vi "Main.vi"(11 "Module Admin":refnum<class "Delacor_lib_QMH_Module Admin.lvclass">) -> ()   [LabVIEW 2019, in "Helper loop.lvlib"]
doc: "This template is based off of the Queued Message Handler design pattern and the Queued Message Handler project template that ships with LabVIEW.\n\nThe main difference is that the queue is private to this module and communication between modules is performed via Broadcast and Request events.\n\nRequest events are wrapped in public API methods and are handled in the Event Handling Loop (EHL) of this VI. Any module can register for Broadcast events sent by this module. The EHL generates messages based on user interface actions.\n\nThe Message Handling Loop (MHL) processes messages generated by the EHL, or by other messages. The messages are string values, so new messages can be added easily to the Message Cases case structure in the MHL. Each message cluster can also provide an optional value for Message Data, which is a variant that can be converted to whatever message-specific data is required.\n_____\nBased on Delacor QMH Project Template 5.0.0.82."
uses:
  Helper loop.lvlib
  Module Data--cluster.ctl
  <vilib>/Delacor/Delacor QMH/Libraries/Message Queue_class/Delacor_lib_QMH_Message Queue.lvclass
  <vilib>/Delacor/Delacor QMH/Libraries/Message Queue_class/Delacor_lib_QMH_Enqueue Message (Single).vi
  <vilib>/ErrorRing/Error Ring.xnode
  <vilib>/Utility/error.llb/Error Cluster From Error Code.vi
  Stop Argument--cluster.ctl
  <vilib>/Delacor/Delacor QMH/Libraries/Module Admin_class/Delacor_lib_QMH_Module Admin.lvclass
  <vilib>/Utility/miscctls.llb/LVPointTypeDef.ctl
  STOP_HELPER_LOOP Argument--cluster.ctl
  DQMHSUBPANE/Libraries/HELPER LOOP ACQ/HELPER LOOP ACQ.lvlib
panel:
  in  "Simulate MHL Error":bool
  in  "Simulate EHL Error":bool
  out "error out":errorcluster
  out "Status":string
  # "Other QMH Modules communicate with this Module via its Public API (wrappers for its Request Events).\n\nThis Module communicates with other Modules via its Broadcast Events.\nAny module that wants to get these messages, just registers for this module's Broadcast events."
  # "This template is for the Delacor Modified Queued Message Handler design pattern.\n\nSee the block diagram for more information on how to use this template."
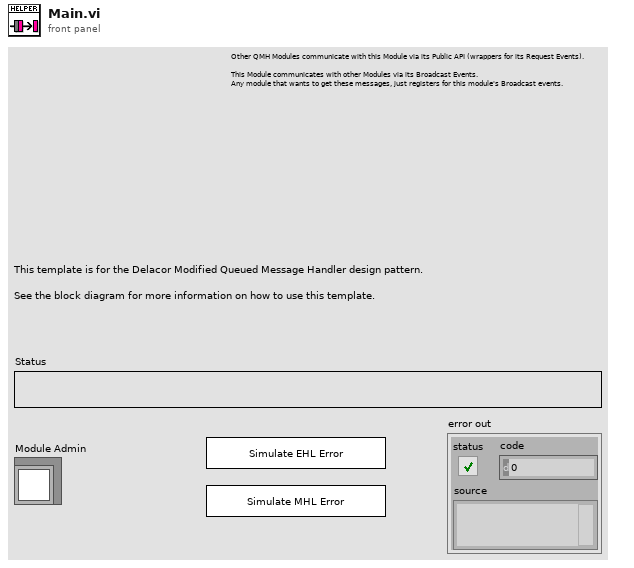
[diagram p1: front panel]
types:
  T1 = typedef "Helper loop.lvlib/Request Events--cluster.ctl" = cluster{"Stop Module":refnum<user-event>, "Show Panel":refnum<user-event>, "Hide Panel":refnum<user-event>, "Get Module Execution Status":refnum<user-event>, "Show Diagram":refnum<user-event>, "START_HELPER_LOOP":refnum<user-event>, "STOP_HELPER_LOOP":refnum<user-event>}
  T2 = typedef "Helper loop.lvlib/Module Data--cluster.ctl" = cluster{"Status":string}
  T3 = typedef "Helper loop.lvlib/STOP_HELPER_LOOP Argument--cluster.ctl" = cluster{"Boolean":bool}
  T4 = enum32{"invalid lock state", "Not Locked", "Locked (No Password)", "Password-protected"}
  T5 = typedef "Helper loop.lvlib/Stop Argument--cluster.ctl" = cluster{"Origin":string, "Exit via Stop Module Req?":bool, "Wait for Module to stop?":bool}
  T6 = typedef "LVPointTypeDef.ctl" = cluster{"Horizontal":i16, "Vertical":i16}
  T7 = enum32{"Invalid", "Standard", "Closed", "Hidden", "Minimized", "Maximized"}
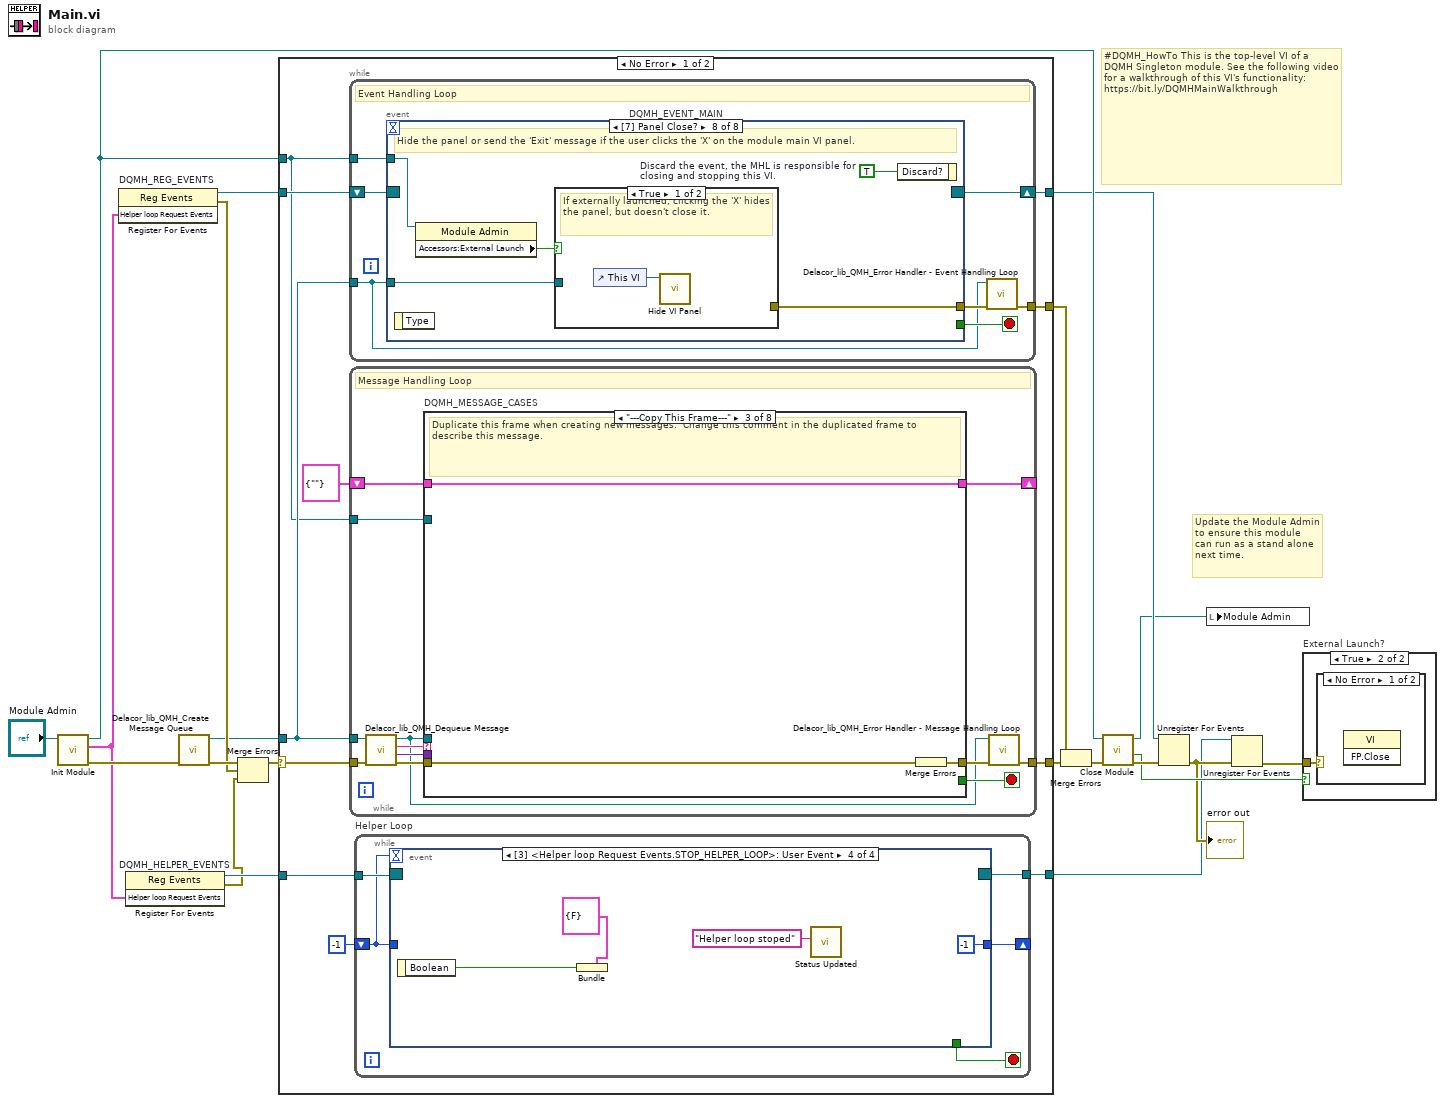
[diagram p0: block diagram]
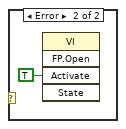
[diagram p3: hidden frame]
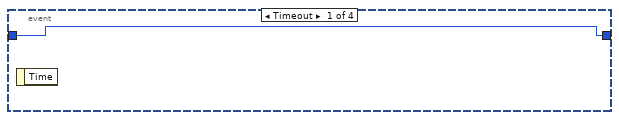
[diagram p4: hidden frame]
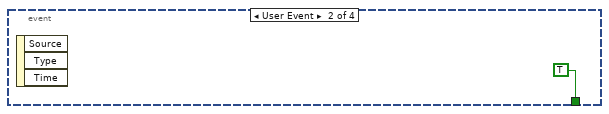
[diagram p5: hidden frame]
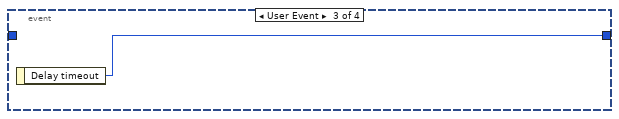
[diagram p6: hidden frame]
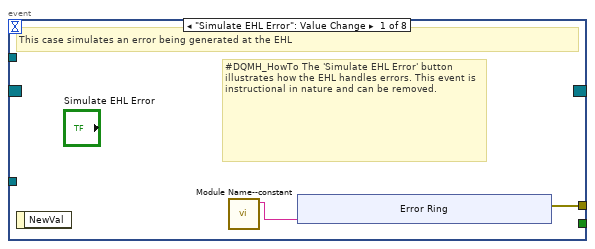
[diagram p7: hidden frame]
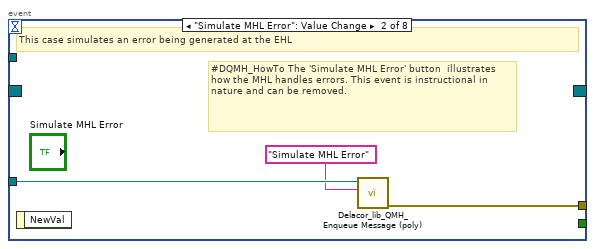
[diagram p8: hidden frame]
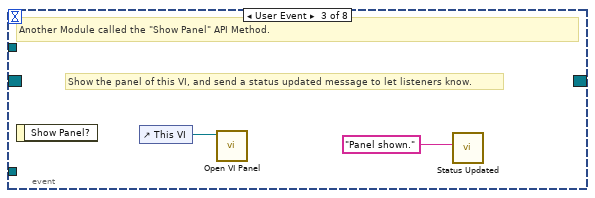
[diagram p9: hidden frame]
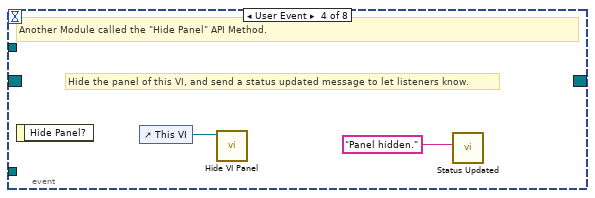
[diagram p10: hidden frame]
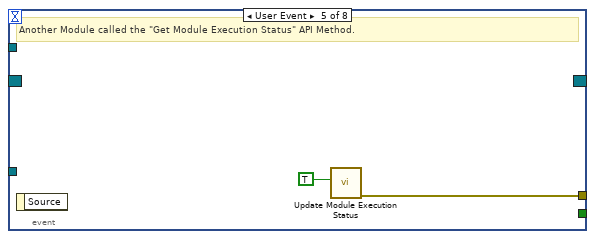
[diagram p11: hidden frame]
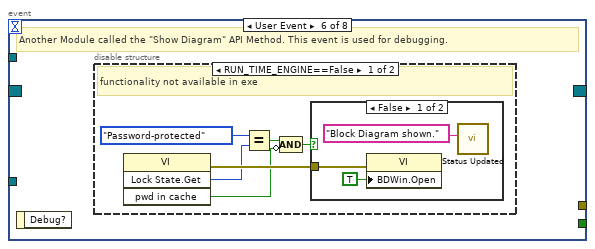
[diagram p12: hidden frame]
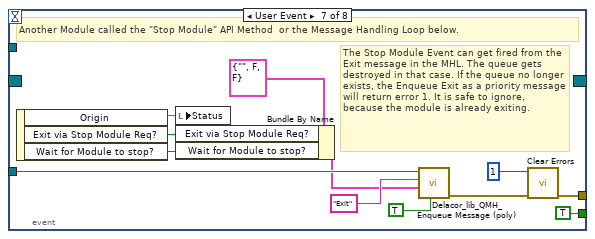
[diagram p15: hidden frame]
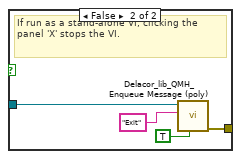
[diagram p16: hidden frame]
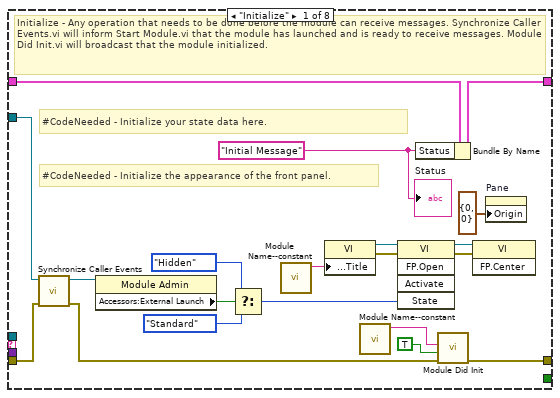
[diagram p17: hidden frame]
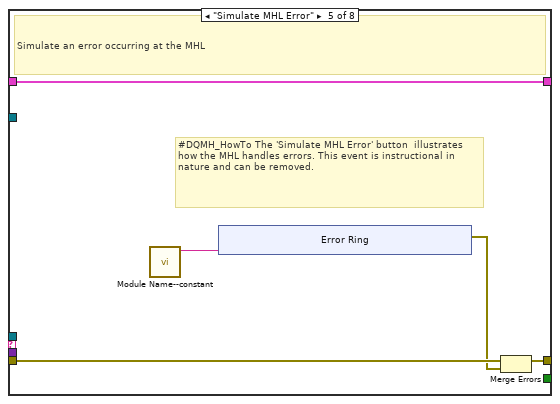
[diagram p20: hidden frame]
diagram:
  # "#DQMH_HowTo This is the top-level VI of a DQMH Singleton module. See the following video for a walkthrough of this VI's functionality: https://bit.ly/DQMHMainWalkthrough"
  # "Update the Module Admin to ensure this module can run as a stand alone next time."
  n1 = call "Init Module.vi"("Singleton Module Admin in"="Module Admin") -> ("error out"=w20:errorcluster, "Helper loop Request Events"=w6:T1, "Singleton Module Admin out"=w13:refnum<class "Delacor_lib_QMH_Module Admin.lvclass">)  [unwired: 8 in]
  n2 = register-events "DQMH_REG_EVENTS"(w6) -> (reference out=w11:refnum<event-registration>, error out=w14:errorcluster)  [unwired: 2 in]
  n3 = register-events "DQMH_HELPER_EVENTS"(w6) -> (reference out=w5:refnum<event-registration>, error out=w4:errorcluster)  [unwired: 2 in]
  n4 = call <vilib>:"Delacor_lib_QMH_Create Message Queue.vi"("error in (no error)"=w20) -> ("error out"=w16:errorcluster, "Message Queue"=w10:refnum<class "Delacor_lib_QMH_Message Queue.lvclass">)  [unwired: 9 in]
  n5 = Merge Errors(w16, w14, w4) -> (w15:errorcluster)
  n6 = case shown="No Error" w15 {
    selector: w15 -> [w30 w201]
    tunnel: [w32 w200] -> w21
    tunnel: [w29 w206] -> w12
    tunnel: w11 -> [w27 w206]
    tunnel: w10 -> [w26 w199]
    tunnel: [w31 _] -> w18
    tunnel: w13 -> [w25 w202]
    tunnel: w5 -> [w24 w198]
    tunnel: [w23 w198] -> w1
    frame No Error {
      n7 = while {
        tunnel: w26 -> [w45]
        shift-right: [w48] -> w29
        shift-left: w27 -> [w49]
        tunnel: [w50] -> w31
        tunnel: w25 -> [w46]
        stop <- w47 stop-if-true
        # "Event Handling Loop"
        n8 = event "DQMH_EVENT_MAIN" shown="[7] Panel Close?" {
          selector: w49 -> [_ _ _ _ _ _ _ _]
          dyn-events: [_ _ _ _ _ _ _ _] -> w48
          timeout: _ -> [_ _ _ _ _ _ _ _]
          tunnel: [_ _ _ _ _ _ TRUE ("Discard?") _] -> w47
          tunnel: w45 -> [_ w62 _ _ _ _ w86 w93]
          tunnel: [w53 w63 _ _ w69 _ w89 w95] -> w51
          tunnel: w46 -> [_ _ _ _ _ _ _ w92]
          event "Simulate EHL Error": Value Change {
            # "#DQMH_HowTo The 'Simulate EHL Error' button  illustrates how the EHL handles errors. This event is instructional in nature and can be removed."
            # "This case simulates an error being generated at the EHL"
            n9 = event-data() -> ()  [unwired: 1 in, 1 out]
            n10 = call "Module Name--constant.vi"() -> ("Module Name"=w52:string)  [unwired: 11 in]
            n11 = xnode "Error Ring"("parameter 0"=w52) -> ("error out"=w53:errorcluster)
          }
          event "Simulate MHL Error": Value Change {
            # "#DQMH_HowTo The 'Simulate MHL Error' button  illustrates how the MHL handles errors. This event is instructional in nature and can be removed."
            # "This case simulates an error being generated at the EHL"
            n12 = event-data() -> ()  [unwired: 1 in, 1 out]
            n13 = call-poly <vilib>:"Delacor_lib_QMH_Enqueue Message (poly).vi"("Message"="Simulate MHL Error", "Message Queue in"=w62) -> ("error out"=w63:errorcluster)  [unwired: 8 in, 1 out]
          }
          event User Event {
            # "Show the panel of this VI, and send a status updated message to let listeners know."
            # "Another Module called the \"Show Panel\" API Method."
            n14 = event-data() -> ()  [unwired: 1 in, 1 out]
            n15 = control-ref of="This VI"() -> (w65:refnum<vi>)
            n16 = call "Open VI Panel.vi"("VI"=w65) -> ()  [unwired: 10 in, 1 out]
            n17 = call "Status Updated.vi"("Status"="Panel shown." ("format string")) -> ()  [unwired: 10 in, 1 out]
          }
          event User Event {
            # "Hide the panel of this VI, and send a status updated message to let listeners know."
            # "Another Module called the \"Hide Panel\" API Method."
            n18 = event-data() -> ()  [unwired: 1 in, 1 out]
            n19 = control-ref of="This VI"() -> (w67:refnum<vi>)
            n20 = call "Hide VI Panel.vi"("VI"=w67) -> ()  [unwired: 10 in, 1 out]
            n21 = call "Status Updated.vi"("Status"="Panel hidden." ("format string")) -> ()  [unwired: 10 in, 1 out]
          }
          event User Event {
            # "Another Module called the \"Get Module Execution Status\" API Method."
            n22 = event-data() -> ()  [unwired: 1 in, 1 out]
            n23 = call "Update Module Execution Status.vi"("Running?"=TRUE) -> ("error out"=w69:errorcluster)  [unwired: 10 in]
          }
          event User Event {
            # "Another Module called the \"Show Diagram\" API Method. This event is used for debugging."
            n24 = event-data() -> ()  [unwired: 1 in, 1 out]
            n25 = disable-structure shown="RUN_TIME_ENGINE==False" {
              frame condition #0 (active) {
                # "functionality not available in exe"
                n26 = invoke class="VI" method="Lock State.Get"() -> (error out=w75:errorcluster, "Get Lock State"=w74:T4, "pwd in cache"=w71:bool)  [unwired: 4 in, 1 out]
                n27 = Equal?(x=T4."Password-protected", y=w74) -> (x = y?=w72:bool)
                n28 = Compound Arithmetic op=AND(w72, invert w71) -> (w70:bool)
                n29 = case shown="False" w70 {
                  tunnel: w75 -> [w78 _]
                  frame False {
                    n30 = property class="VI"(error in=w78, "BDWin.Open"=TRUE ("Block Diagram Window:Open")) -> ()  [unwired: 1 in, 2 out]
                    n31 = call "Status Updated.vi"("Status"="Block Diagram shown." ("format string")) -> ()  [unwired: 10 in, 1 out]
                  }
                  frame True {
                    # "Password-protected VI, and the password is not in the cache. Do not show the diagram."
                  }
                }
              }
              frame condition #1 {
              }
            }
          }
          event User Event {
            # "The Stop Module Event can get fired from the Exit message in the MHL. The queue gets destroyed in that case. If the queue no longer exists, the Enqueue Exit as a priority message will return error 1. It is safe to ignore, because the module is already exiting."
            # "Another Module called the \"Stop Module\" API Method  or the Message Handling Loop below."
            n32 = event-data() -> ("Origin"=w85:string, "Exit via Stop Module Req?"=w81:bool, "Wait for Module to stop?"=w80:bool)  [unwired: 1 in]
            n33 = local write "Status"(w85) -> ()
            n34 = Bundle By Name(cluster=T5 {"Origin"="", "Exit via Stop Module Req?"=FALSE, "Wait for Module to stop?"=FALSE} ("Stop Argument"), "Exit via Stop Module Req?"=w81, "Wait for Module to stop?"=w80) -> (w79:T5)
            n35 = call-poly <vilib>:"Delacor_lib_QMH_Enqueue Message (poly).vi"("Priority Message? (F)"=TRUE, "Message Data"=w79, "Message"="Exit", "Message Queue in"=w86) -> ("error out"=w90:errorcluster)  [unwired: 6 in, 1 out]
            n36 = call <vilib>:"Clear Errors.vi"("error in (no error)"=w90, "specific error code to clear (0: all)"=1) -> ("error out"=w89:errorcluster)  [unwired: 4 in, 1 out]
          }
          event Panel Close? {
            w94 = TRUE  # Discard the event, the MHL is responsible for closing and stopping this VI.
            # "Hide the panel or send the 'Exit' message if the user clicks the 'X' on the module main VI panel."
            n37 = event-data() -> ()  [unwired: 1 in, 1 out]
            n38 = property class="Module Admin"(reference=w92) -> ("Accessors:External Launch"=w91:bool)  [unwired: 1 in, 2 out]
            n39 = case shown="True" w91 {
              tunnel: w93 -> [_ w99]
              tunnel: [_ w100] -> w95
              frame True {
                # "If externally launched, clicking the 'X' hides the panel, but doesn't close it."
                n40 = control-ref of="This VI"() -> (w96:refnum<vi>)
                n41 = call "Hide VI Panel.vi"("VI"=w96) -> ()  [unwired: 10 in, 1 out]
              }
              frame False {
                # "If run as a stand-alone VI, clicking the panel 'X' stops the VI."
                n42 = call-poly <vilib>:"Delacor_lib_QMH_Enqueue Message (poly).vi"("Priority Message? (F)"=TRUE, "Message"="Exit", "Message Queue in"=w99) -> ("error out"=w100:errorcluster)  [unwired: 7 in, 1 out]
              }
            }
            n43 = event-data("Discard?"=w94) -> ()  [unwired: 1 in, 1 out]
          }
        }
        n44 = call-dynamic "Delacor_lib_QMH_Error Handler - Event Handling Loop.vi"("error in (no error)"=w51, "Message Queue in"=w45) -> ("dup error in"=w50:errorcluster)  [unwired: 8 in, 1 out]
      }
      n45 = while {
        tunnel: w26 -> [w103]
        shift-right: [w107] -> _
        shift-left: T2 {"Status"=""} ("Data Cluster") -> [w108]
        tunnel: w30 -> [w111]
        tunnel: [w109] -> w32
        tunnel: w25 -> [w101]
        stop <- w106 stop-if-true
        # "Message Handling Loop"
        n46 = call-dynamic "Delacor_lib_QMH_Dequeue Message.vi"("error in (no error)"=w111, "Message Queue in"=w103) -> ("error out"=w110:errorcluster, "Message Data"=w104:variant, "Message"=w105:string, "Message Queue out"=w102:refnum<class "Delacor_lib_QMH_Message Queue.lvclass">)  [unwired: 6 in]
        n47 = case "DQMH_MESSAGE_CASES" shown="\"---Copy This Frame---\"" w105 {
          selector: w105 -> [_ _ _ _ _ _ _ w185]
          tunnel: w102 -> [_ _ _ _ _ w155 w177 _]
          tunnel: w110 -> [w130 w134 w137 w139 w144 w162 w183 w187]
          tunnel: [w128 w134 w136 w139 w143 w158 w180 w188] -> w112
          tunnel: w108 -> [w119 w133 w135 w138 w141 w157 w176 w186]
          tunnel: [w118 w133 w135 w138 w141 w157 w176 w186] -> w107
          tunnel: [_ _ _ _ _ _ w175 _] -> w106
          tunnel: w104 -> [_ _ _ _ _ w156 w174 _]
          tunnel: w101 -> [w120 _ _ _ _ w154 w169 _]
          frame "Initialize" {
            w113 = "Initial Message" ("Initial Message")
            # "#CodeNeeded - Initialize the appearance of the front panel."
            # "#CodeNeeded - Initialize your state data here."
            # "Initialize - Any operation that needs to be done before the module can receive messages. Synchronize Caller Events.vi will inform Start Module.vi that the module has launched and is ready to receive messages. Module Did Init.vi will broadcast that the module initialized."
            n48 = call "Synchronize Caller Events.vi"("error in (no error)"=w130, "Singleton Module Admin in"=w120) -> ("error out"=w129:errorcluster, "Singleton Module Admin out"=w115:refnum<class "Delacor_lib_QMH_Module Admin.lvclass">)  [unwired: 8 in]
            n49 = property class="Module Admin"(reference=w115) -> ("Accessors:External Launch"=w124:bool)  [unwired: 1 in, 2 out]
            n50 = Select(t=T7."Hidden" ("State"), s=w124, f=T7."Standard" ("State")) -> (s? t:f=w121:T7)
            n51 = call "Module Name--constant.vi"() -> ("Module Name"=w127:string)  [unwired: 11 in]
            n52 = property class="VI"("Front Panel.Title"=w127) -> (reference out=w126:refnum<vi>, error out=w132:errorcluster)  [unwired: 2 in]
            n53 = call "Module Name--constant.vi"() -> ("Module Name"=w116:string)  [unwired: 11 in]
            n54 = invoke class="VI" method="FP.Open"(reference=w126, error in=w132, "State"=w121) -> (reference out=w125:refnum<vi>, error out=w131:errorcluster)  [unwired: 2 in, 3 out]
            n55 = Bundle By Name(cluster=w119, "Status"=w113) -> (w118:T2)
            n56 = call "Module Did Init.vi"("error in (no error)"=w129, "Initialized?"=TRUE, "Origin"=w116) -> ("error out"=w128:errorcluster)  [unwired: 8 in]
            n57 = invoke class="VI" method="FP.Center"(reference=w125, error in=w131) -> ()  [unwired: 1 in, 3 out]
            n58 = property on="Pane" class="Pane"("Origin"=T6 {"Horizontal"=0, "Vertical"=0}) -> ()  [unwired: 2 in, 2 out]
            "Status" <- w113
          }
          frame "--- Module Specific ---" {
            # "Separator -- The following cases handle messages specific to this Module."
          }
          frame "---Copy This Frame---" {
            # "Duplicate this frame when creating new messages.  Change this comment in the duplicated frame to describe this message."
            n59 = Merge Errors(w137) -> (w136:errorcluster)
          }
          frame "--- Exit and Error Handling---" {
            # "Separator - The following cases handle errors and exit messages."
          }
          frame "Simulate MHL Error" {
            # "#DQMH_HowTo The 'Simulate MHL Error' button  illustrates how the MHL handles errors. This event is instructional in nature and can be removed."
            # "Simulate an error occurring at the MHL"
            n60 = call "Module Name--constant.vi"() -> ("Module Name"=w140:string)  [unwired: 11 in]
            n61 = xnode "Error Ring"("parameter 0"=w140) -> ("error out"=w142:errorcluster)
            n62 = Merge Errors(w144, w142) -> (w143:errorcluster)
          }
          frame "Error" {
            # "#CodeRecommended - If you ever change the name of this \"Error\" message, you'll need to update the name in the Check Loop Error.vi as well."
            # "#CodeRecommended - If the module is running in standalone mode (External Launch = FALSE), this code will pop up an error dialog and call the 'Exit' message if an error occurs. Add more fine-grained error handling here."
            # "Error - Check the error message data and respond accordingly. This message is sent by the \"Error Handler\" VIs at the end of each loop in this application."
            n63 = property class="Module Admin"(reference=w154) -> ("Accessors:External Launch"=w153:bool)  [unwired: 1 in, 2 out]
            n64 = Variant To Data(error in=w162, type=errorcluster {"status"=FALSE, "code"=0, "source"=""} ("error constant"), Variant=w156) -> (data=w163:errorcluster, error out=w160:errorcluster)
            n65 = call "Module Name--constant.vi"() -> ("Module Name"=w152:string)  [unwired: 11 in]
            n66 = call "Error Reported.vi"("Additional Information"=w152, "Error"=w163) -> ()  [unwired: 9 in, 1 out]
            n67 = case shown="False" w153 {
              tunnel: [w168 _] -> w159
              tunnel: w155 -> [w166 _]
              tunnel: w163 -> [w167 _]
              frame False {
                # "If the module is running standalone, then pop up an error dialog and call the \"Exit\" message."
                n68 = call <vilib>:"Simple Error Handler.vi"("error in (no error)"=w167) -> ()  [unwired: 4 in, 5 out]
                n69 = call-poly <vilib>:"Delacor_lib_QMH_Enqueue Message (poly).vi"("Priority Message? (F)"=TRUE, "Message"="Exit", "Message Queue in"=w166) -> ("error out"=w168:errorcluster)  [unwired: 7 in, 1 out]
              }
              frame True {
                # "If the module was launched externally, calling the Error Reported broadcast VI is the only action performed by the \"Error\" message. The module's caller can then process the error appropriately."
              }
            }
            n70 = Merge Errors(w160, w159) -> (w158:errorcluster)
            n71 = local write "error out"(w158) -> ()
          }
          frame "Exit" {
            w173 = 91  # 91: not all Exit messages will have an argument
            w175 = TRUE  # Stop the VI
            # "Release the message queue reference"
            # "#CodeNeeded - Add any required cleanup code here"
            # "Exit - Exit the application."
            n72 = Variant To Data(error in=w183, type=T5 {"Origin"="", "Exit via Stop Module Req?"=FALSE, "Wait for Module to stop?"=FALSE} ("Stop Argument"), Variant=w174) -> (data=w171:T5, error out=w179:errorcluster)
            n73 = call <vilib>:"Clear Errors.vi"("error in (no error)"=w179, "specific error code to clear (0: all)"=w173) -> ("error out"=w182:errorcluster)  [unwired: 4 in, 1 out]
            n74 = control-ref of="This VI"() -> (w170:refnum<vi>)
            n75 = call-dynamic "Delacor_lib_QMH_Release Message Queue.vi"("error in (no error)"=w182, "Message Queue"=w177) -> ("error out"=w181:errorcluster)  [unwired: 9 in]
            n76 = call "Handle Exit.vi"("Stop Argument"=w171, "Admin in"=w169, "VI reference"=w170) -> ("error out"=w178:errorcluster)  [unwired: 7 in, 1 out]
            n77 = Merge Errors(w181, w178) -> (w180:errorcluster)
          }
          frame Default {
            # "'Default' case only runs if there is a message that isn't defined in any of the other cases.  Output a programming error."
            n78 = call "Module Name--constant.vi"() -> ("Module Name"=w184:string)  [unwired: 11 in]
            n79 = xnode "Error Ring"("parameter 0"=w185, "parameter 1"=w184) -> ("error out"=w189:errorcluster)
            n80 = Merge Errors(w187, w189) -> (w188:errorcluster)
          }
        }
        n81 = call-dynamic "Delacor_lib_QMH_Error Handler - Message Handling Loop.vi"("error in (no error)"=w112, "Message Queue in"=w102) -> ("dup error in"=w109:errorcluster)  [unwired: 8 in, 1 out]
      }
      n82 = while "Helper Loop" {
        tunnel: w24 -> [w37]
        tunnel: [w36] -> w23
        shift-right: [w35] -> _
        shift-left: -1 ("Delay timeout") -> [w34]
        stop <- w33 stop-if-true
        n83 = event shown="[3] <Helper loop Request Events.STOP_HELPER_LOOP>: User Event" {
          selector: w37 -> [_ _ _ _]
          dyn-events: [_ _ _ _] -> w36
          timeout: w34 -> [_ _ _ _]
          tunnel: [w38 _ w40 -1 ("Delay timeout")] -> w35
          tunnel: w34 -> [w38 _ _ _]
          tunnel: [_ TRUE _ _] -> w33
          event Timeout {
            n84 = event-data() -> ()  [unwired: 1 in, 1 out]
          }
          event User Event {
            n85 = event-data() -> ()  [unwired: 1 in, 3 out]
          }
          event User Event {
            n86 = event-data() -> ("Delay timeout"=w40:i32)  [unwired: 1 in]
          }
          event User Event {
            n87 = event-data() -> ("Boolean"=w44:bool)  [unwired: 1 in]
            n88 = Bundle(cluster=T3 {"Boolean"=FALSE} ("STOP_HELPER_LOOP Argument"), "Boolean"=w44) -> ()  [unwired: 1 out]
            n89 = call "Status Updated.vi"("Status"="Helper loop stoped") -> ()  [unwired: 10 in, 1 out]
          }
        }
      }
    }
    frame Error {
      # "Synchronize Caller Events.vi will inform Start Module.vi that the module has launched and will let the code calling Start Module.vi register for broadcasts and would permit the caller receive the broadcast that an error occurred at launch time."
      n90 = call-dynamic "Delacor_lib_QMH_Release Message Queue.vi"("error in (no error)"=w201, "Message Queue"=w199) -> ("error out"=w200:errorcluster)  [unwired: 9 in]
      n91 = call "Synchronize Caller Events.vi"("Singleton Module Admin in"=w202) -> ("error out"=w207:errorcluster)  [unwired: 9 in, 1 out]
      n92 = call "Module Name--constant.vi"() -> ("Module Name"=w205:string)  [unwired: 11 in]
      n93 = Format Into String(format string="An error occurred during initialization. %s is no longer running.", w205) -> (resulting string=w203:string)  [unwired: 2 in, 1 out]
      n94 = Merge Errors(w200, w207) -> (w208:errorcluster)
      n95 = call "Error Reported.vi"("Additional Information"=w203, "Error"=w208) -> ()  [unwired: 9 in, 1 out]
    }
  }
  n96 = Merge Errors(w18, w21) -> (w17:errorcluster)
  n97 = call "Close Module.vi"("error in (no error)"=w17, "Module Admin in"=w13) -> ("error out"=w19:errorcluster, "External Launch"=w7:bool, "Module Admin out"=w8:refnum<class "Delacor_lib_QMH_Module Admin.lvclass">)  [unwired: 7 in]
  n98 = Unregister For Events(event registration refnum=w12, error in=w19) -> (error out=w3:errorcluster)
  "error out" <- w3
  n99 = local write "Module Admin"(w8) -> ()
  n100 = Unregister For Events(event registration refnum=w1, error in=w3) -> (error out=w2:errorcluster)
  n101 = case "External Launch?" shown="True" w7 {
    tunnel: w2 -> [_ w209]
    frame False {
    }
    frame True {
      n102 = case shown="No Error" w209 {
        frame No Error {
          n103 = invoke class="VI" method="FP.Close"() -> ()  [unwired: 3 in, 3 out]
        }
        frame Error {
          n104 = invoke class="VI" method="FP.Open"("Activate"=TRUE ("Activate?")) -> ()  [unwired: 4 in, 5 out]
        }
      }
    }
  }
